vi "Actor Core.vi"(8 "error in":errorcluster, 11 "Timing Engine Tester in":refnum<class "Timing Engine Tester.lvclass">) -> (0 "error out":errorcluster, 3 "Actor out":refnum<class "Actor.lvclass">)   [LabVIEW 2016, in "Assert API Components.lvlib" / "Assert Display.lvlib" / "Timing Engine Tester.lvlib" / "Timing Engine Tester.lvclass"]
doc: "(<B>Filename</B>: Actor Framework.lvlib:Actor.lvclass:Actor Core.vi)\n\nReceives messages to the actor, reacts to them, and initiates any error handling that may shut the actor down.\n\nDescendant classes may override this VI to append parallel tasks for the actor to complete while it handles messages. Overrides use the Call Parent Method node."
uses:
  Timing Engine Tester.lvclass
  C:/Program Files (x86)/National Instruments/LabVIEW 2016/vi.lib/ActorFramework/Actor/Actor.lvclass
  <vilib>/ActorFramework/Actor/Actor.lvclass
  Core/Timing Engine/Timing Engine/Timing Engine.lvclass
  Timing Engine Tester Messages/Generate Test Event Msg/Generate Test Event Msg.lvclass
  C:/Users/ukhornp/Documents/Projects/actor_assert_api/Core/Timing Engine/Timing Engine Messages/Update Msg/Update Msg.lvclass
  Core/Timing Engine/Timing Engine/Timing Engine.lvclass/Timing Engine.ctl
  <vilib>/ActorFramework/Actor/Actor.lvclass/Actor.ctl
  <vilib>/ActorFramework/Message Enqueuer/Message Enqueuer.lvclass/Message Enqueuer.ctl
  Timing Engine Tester.lvclass/Timing Engine Tester.ctl
  <vilib>/ActorFramework/Message Enqueuer/Init from Existing Queue.vi
  <vilib>/ActorFramework/Message Enqueuer/Enqueue.vi
  <vilib>/ActorFramework/Stop Msg/Stop Msg.lvclass
  C:/Program Files (x86)/National Instruments/LabVIEW 2016/vi.lib/ActorFramework/Message/Message.lvclass
  <vilib>/Utility/LVClass/Get LV Class Name.vi
  <resource>/AFDebug/Generate Trace for Message.vi
  <vilib>/ActorFramework/Message Priority Queue/Priority Enqueue.vi
  <vilib>/ActorFramework/Message Enqueuer/Message Enqueuer.lvclass
panel:
  out "Count":i32
  in  "stop":bool
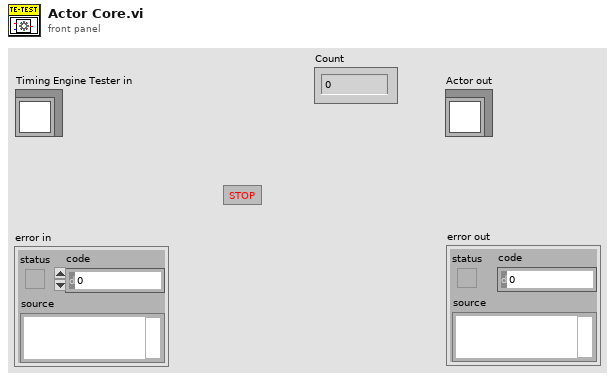
[diagram p1: front panel]
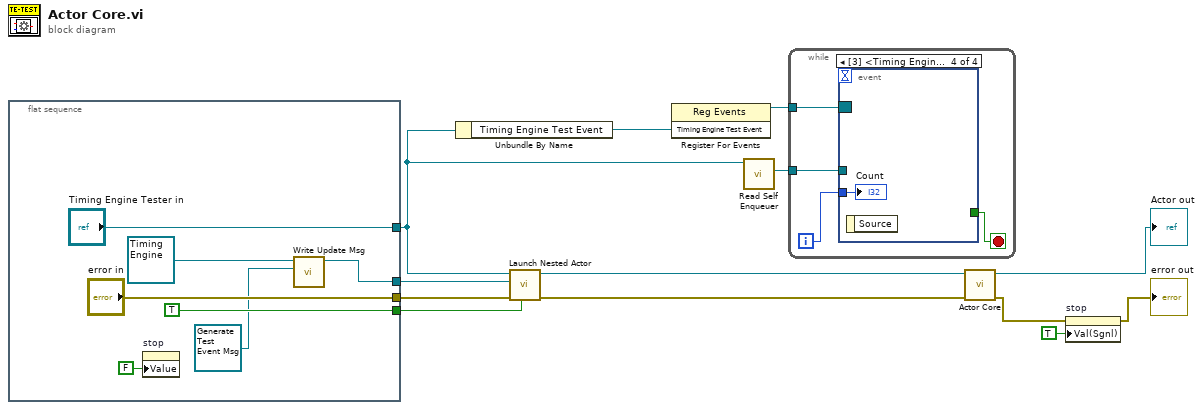
[diagram p0: block diagram]
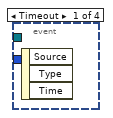
[diagram p2: hidden frame]
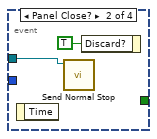
[diagram p3: hidden frame]
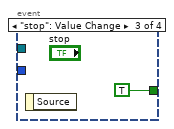
[diagram p4: hidden frame]
diagram:
  n1 = flat-sequence {
    tunnel: ["error in"] -> w12
    tunnel: [TRUE ("Open Actor Core front panel? (F)")] -> w9
    tunnel: [w15] -> w8
    tunnel: ["Timing Engine Tester in"] -> w3
    frame #0 {
      n2 = property on="stop" class="Bool (strict)"("Value"=FALSE ("stop")) -> ()  [unwired: 2 in, 2 out]
      n3 = call "Write Update Msg.vi"("Assert API Components.lvlib:Assert Display.lvlib:Timing Engine.lvlib:Update Msg.lvclass"=refnum<class "Generate Test Event Msg.lvclass"> refnum ("Assert API Components.lvlib:Assert Display.lvlib:Timing Engine Tester.lvlib:Generate Test Event Msg.lvclass"), "Timing Engine in"=refnum<class "Timing Engine.lvclass"> refnum ("Assert API Components.lvlib:Assert Display.lvlib:Timing Engine.lvlib:Timing Engine.lvclass")) -> ("Timing Engine out"=w15:refnum<class "Timing Engine.lvclass">)  [unwired: 9 in]
    }
  }
  n4 = Unbundle By Name(w3) -> ("Timing Engine Test Event"=w2:refnum<user-event>)
  n5 = call <vilib>:"Launch Nested Actor.vi"("Open Actor Core front panel? (F)"=w9, "error in (no error)"=w12, "Nested Actor"=w8, "Caller Actor in"=w3) -> ("error out"=w11:errorcluster, "Caller Actor out"=w10:refnum<class "Timing Engine Tester.lvclass">)  [unwired: 5 in, 1 out]
  n6 = register-events(w2) -> (reference out=w1:refnum<event-registration>)  [unwired: 2 in, 1 out]
  n7 = call <vilib>:"Read Self Enqueuer.vi"("Actor"=w3) -> ("Self Enqueuer"=w7:refnum<class "Message Enqueuer.lvclass">)  [unwired: 10 in]
  n8 = while {
    tunnel: w7 -> [w24]
    tunnel: w1 -> [w21]
    i -> [w22]
    stop <- w23 stop-if-true
    n9 = event shown="[3] <Timing Engine Test Event>: User Event" {
      selector: w21 -> [_ _ _ _]
      dyn-events: _ -> [_ _ _ _]
      timeout: _ -> [_ _ _ _]
      tunnel: w24 -> [_ w25 _ _]
      tunnel: [_ _ TRUE _] -> w23
      tunnel: w22 -> [_ _ _ w28]
      event Timeout {
        n10 = event-data() -> ()  [unwired: 1 in, 3 out]
      }
      event Panel Close? {
        n11 = event-data() -> ()  [unwired: 1 in, 1 out]
        n12 = call <vilib>:"Send Normal Stop.vi"("Message Enqueuer"=w25) -> ()  [unwired: 10 in, 1 out]
        n13 = event-data("Discard?"=TRUE) -> ()  [unwired: 1 in, 1 out]
      }
      event "stop": Value Change {
        n14 = event-data() -> ()  [unwired: 1 in, 1 out]
      }
      event User Event {
        n15 = event-data() -> ()  [unwired: 1 in, 1 out]
        "Count" <- w28
      }
    }
  }
  n16 = call-parent "Actor Core.vi"("error in"=w11, "Actor in"=w10) -> ("error out"=w5:errorcluster, "Actor out"=→"Actor out":refnum<class "Actor.lvclass">)  [unwired: 8 in]
  n17 = property on="stop" class="Bool (strict)"(error in=w5, "Val(Sgnl)"=TRUE ("Value (Signaling)")) -> (error out=→"error out":errorcluster)  [unwired: 1 in, 1 out]
